vi "Open Arms.vi"(8 "error in (no error)":errorcluster, 11 "Dev Grabber in":refnum<class "Dev Grabber.lvclass">) -> (0 "error out":errorcluster, 3 "Dev Grabber out":refnum<class "Dev Grabber.lvclass">)   [LabVIEW 2014, in "Dev Grabber.lvlib" / "Dev Grabber.lvclass"]
uses:
  Dev Grabber.lvclass
  <vilib>/Rock Robotics/WPI/Solenoid/WPI_SolenoidValue.ctl
  Dev Grabber.lvclass/Dev Grabber.ctl
  <vilib>/Rock Robotics/WPI/Solenoid/WPI_SolenoidSetEnum.vi
  Robot/Grabber/Grabber Class/Grabber.lvclass
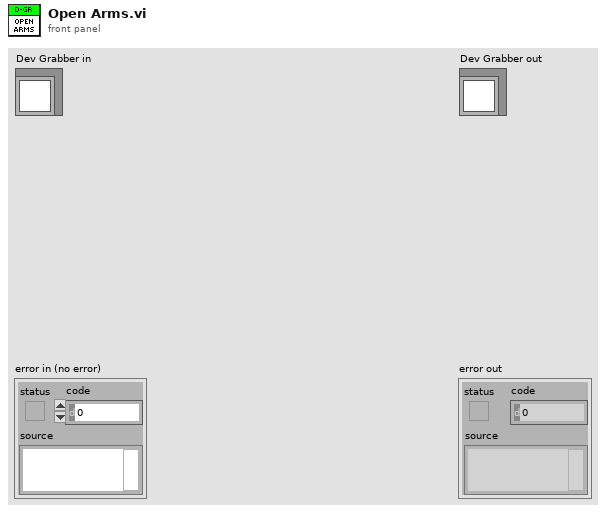
[diagram p1: front panel]
types:
  T1 = typedef "WPI_SolenoidValue.ctl" = enum16{"Off", "On", "Forward", "Reverse"}
  T2 = typedef "WPI_SolenoidDevRef.ctl" = cluster{"DevStatus":errorcluster, "Pneumatics Control Module":u8, "Forward Solenoid Channel":T3, "Reverse Solenoid Channel":T3}
  T3 = typedef "WPI_SolenoidChannel.ctl" = enum8{"Solenoid 0", "Solenoid 1", "Solenoid 2", "Solenoid 3", "Solenoid 4", "Solenoid 5", "Solenoid 6", "Solenoid 7", "Invalid"}
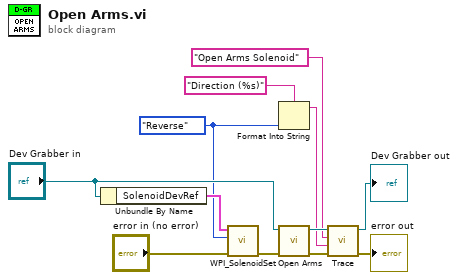
[diagram p0: block diagram]
diagram:
  w2 = WPI_SolenoidValue."Reverse" ("Value")
  n1 = Unbundle By Name("Dev Grabber in") -> ("SolenoidDevRef"=w11:T2)
  n2 = call-poly <vilib>:"WPI_SolenoidSet.vi"("error in (no error)"="error in (no error)", "Value"=w2, "SolenoidDevRef"=w11) -> ("error out"=w9:errorcluster)  [unwired: 7 in, 1 out]
  n3 = Format Into String(format string="Direction (%s)", w2) -> (resulting string=w1:string)  [unwired: 2 in, 1 out]
  n4 = call-parent "Open Arms.vi"("error in (no error)"=w9, "Grabber in"="Dev Grabber in") -> ("error out"=w8:errorcluster, "Grabber out"=w6:refnum<class "Dev Grabber.lvclass">)  [unwired: 8 in]
  n5 = call-dynamic "Trace.vi"("error in (no error)"=w8, "System Message"=w1, "System Action"="Open Arms Solenoid", "System Actor in"=w6) -> ("error out"=→"error out":errorcluster, "System Actor out"=→"Dev Grabber out":refnum<class "Dev Grabber.lvclass">)  [unwired: 6 in]
